vi "Assert True.vi"(4 "Execution time (s)":dbl=-1.0, 5 "Assert Only? (F)":bool, 6 "error code (1)":i32=1, 7 "Label":string, 8 "error in (no error)":errorcluster, 9 "call chain ignore depth (2)":i32=2, 11 "True?":bool) -> (0 "error out":errorcluster)   [LabVIEW 2013, in "Caraya.lvlib" / "Assert.lvclass"]
doc: "Generates an error if the input condition is not met.\n\n--\nCopyright © 2015 JKI All rights reserved.\n\nAuthor: Tomi Maila <tomi.maila@jki.net>\n\nThis library is provided \"AS IS\" ,WITHOUT WARRANTIES OR\nCONDITIONS OF ANY KIND, either express or implied.\n\nJKI -- jki.net"
uses:
  Assert.lvclass
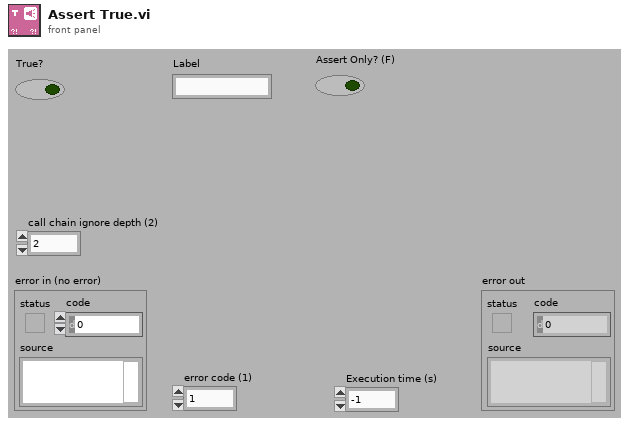
[diagram p1: front panel]
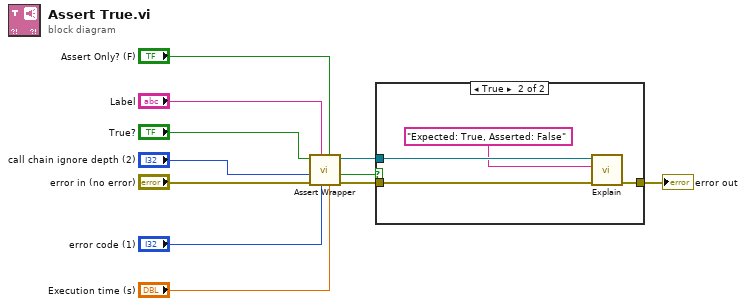
[diagram p0: block diagram]
diagram:
  n1 = call "Assert Wrapper.vi"("Execution time (s)"="Execution time (s)", "Assert Only? (F)"="Assert Only? (F)", "error code (1)"="error code (1)", "Label"="Label", "error in (no error)"="error in (no error)", "call chain ignore depth (2)"="call chain ignore depth (2)", "Assert?"="True?") -> ("error out"=w5:errorcluster, "Verbose"=w3:bool, "Assert out"=w2:refnum<class "Assert.lvclass">)  [unwired: 2 in]
  n2 = case shown="True" w3 {
    tunnel: [w12 w16] -> w7
    tunnel: w2 -> [_ w15]
    tunnel: w5 -> [w12 w14]
    frame False {
    }
    frame True {
      n3 = call "Explain.vi"("error in (no error)"=w14, "Verbose Explanation"="Expected: True, Asserted: False", "Assert in"=w15) -> ("error out"=w16:errorcluster)  [unwired: 7 in, 1 out]
    }
  }
  "error out" <- w7
